vi "GetLine.vi"(8 "error in (no error)":errorcluster caption="Fehler (Eingang, kein Fehler)", 11 "MoveoSerial Eingang":refnum<class "MoveoSerial.lvclass">) -> (0 "error out":errorcluster caption="Fehler (Ausgang)", 2 "RecivedLine":string, 3 "MoveoSerial Ausgang":refnum<class "MoveoSerial.lvclass">)   [LabVIEW 2019, in "MoveoSerial.lvclass"]
uses:
  MoveoSerial.lvclass
  MoveoSerial.lvclass/MoveoSerial.ctl
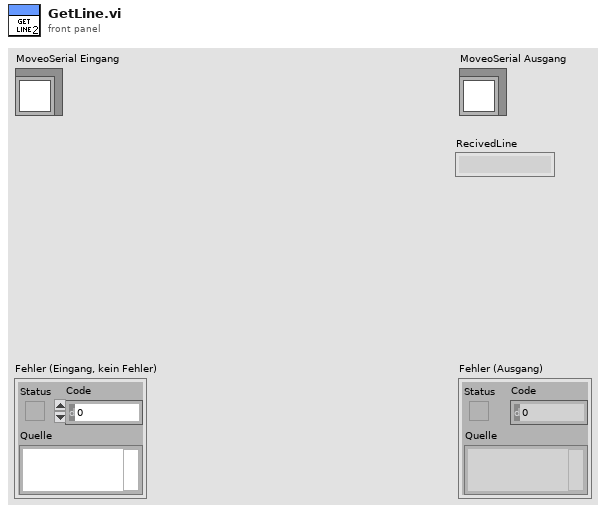
[diagram p1: front panel]
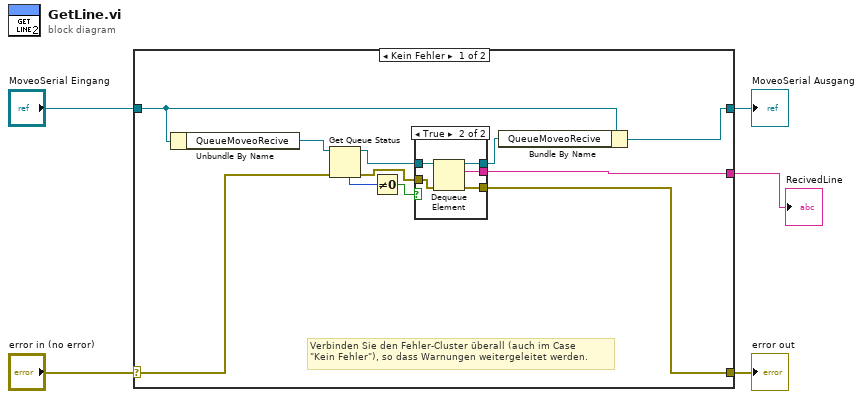
[diagram p0: block diagram]
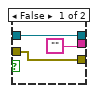
[diagram p2: hidden frame]
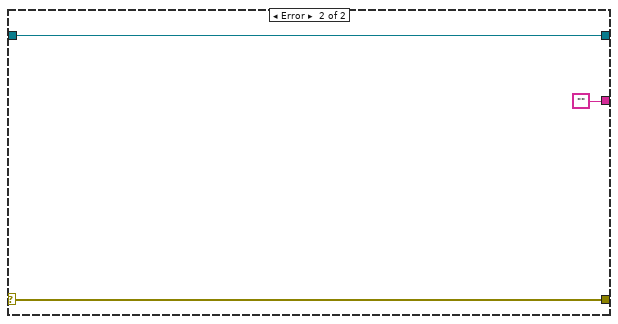
[diagram p3: hidden frame]
diagram:
  n1 = case shown="Kein Fehler" "error in (no error)" {
    selector: "error in (no error)" -> [w10 w27]
    tunnel: [w16 w27] -> w4
    tunnel: [w14 w26] -> w2
    tunnel: "MoveoSerial Eingang" -> [w15 w26]
    tunnel: [w12 ""] -> w1
    frame No Error {
      # "Verbinden Sie den Fehler-Cluster überall (auch im Case\n\"Kein Fehler\"), so dass Warnungen weitergeleitet werden."
      n2 = Unbundle By Name(w15) -> ("QueueMoveoRecive"=w11:refnum<queue>)
      n3 = Get Queue Status(queue=w11, error in (no error)=w10) -> (queue out=w8:refnum<queue>, error out=w6:errorcluster, # elements in queue=w9:i32)  [unwired: 1 in, 5 out]
      n4 = Not Equal To 0?(x=w9) -> (x != 0?=w7:bool)
      n5 = case shown="True" w7 {
        tunnel: [w17 w24] -> w16
        tunnel: [w19 w23] -> w13
        tunnel: ["" w22] -> w12
        tunnel: w8 -> [w19 w21]
        tunnel: w6 -> [w17 w20]
        frame False {
        }
        frame True {
          n6 = Dequeue Element(queue=w21, error in (no error)=w20) -> (queue out=w23:refnum<queue>, element=w22:string, error out=w24:errorcluster)  [unwired: 1 in, 1 out]
        }
      }
      n7 = Bundle By Name(cluster=w15, "QueueMoveoRecive"=w13) -> (w14:refnum<class "MoveoSerial.lvclass">)
    }
    frame Error {
    }
  }
  "error out" <- w4
  "MoveoSerial Ausgang" <- w2
  "RecivedLine" <- w1
